vi "DAQ_E_mIO_DIO.get bit.vi"(0 "i ref in":refnum<vi>, 2 "bitIndex":u32, 3 "ms timeout (10000)":i32=10000, 5 "error in (no error)":errorcluster) -> (14 "i ref out":refnum<vi>, 16 "bit":bool, 17 "timed out":bool, 19 "error out":errorcluster)   [LabVIEW 2014, in "DAQ_E_mIO_DIO.lvlib"]
doc: "Gets a bit from a digital input port\n\nLicense Agreement for this software:\n\nCopyright (C)\nGesellschaft für Schwerionenforschung, GSI\nPlanckstr. 1\n64291 Darmstadt\nGermany\n\nContact: D.Beck@gsi.de \n\nThis program is free software; you can redistribute it and/or modify it under the terms of the GNU General Public License as published by the Free Software Foundation; either version 2 of the license, or (at your option) any later version.\n\nThis program is distributed in the hope that it will be useful, but WITHOUT ANY WARRANTY; without even the implied warranty of MERCHANTABILITY or FITNESS FOR A PARTICULAR PURPOSE. See the GNU General License for more details (http://www.gnu.org).\n\nGesellschaft für Schwerionenforschung, GSI\nPlanckstr. 1, 64291 Darmstadt, Germany\nFor all questions and ideas contact: M.Richter@gsi.de, H.Brand@gsi.de or D.Beck@gsi.de.\nLast update: 17-JUN-2004"
uses:
  DAQ_E_mIO_DIO.lvlib
  CSCore/CSSystem/CoreDefs/CoreDefs.error_type.ctl
  CSApplicationBaseClasses/DigiIOBase/DigiIOBase.directionType.ctl
  CSApplicationBaseClasses/DigiIOBase/DigiIOBase.serviceType.ctl
  lib.lib/UtilityLib/UtilityLib.valueStatus.ctl
  <vilib>/DAQmx/read.llb/DAQmx Read (Digital 1D Bool 1Chan 1Samp).vi
  CSCore/CSSystem/CoreLib/CoreLib.lvlib
  CSApplicationBaseClasses/DigiIOBase/DigiIOBase.lvlib
  lib.lib/UtilityLib/UtilityLib.lvlib
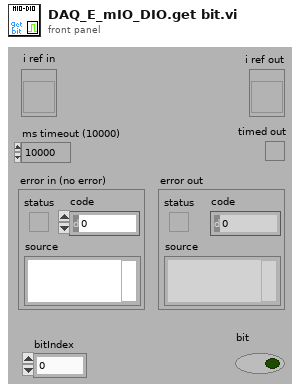
[diagram p1: front panel]
types:
  T1 = typedef "CoreDefs.error_type.ctl" = enum16{"no error", "can't load process", "can't unload process", "process does not exist", "can't install process", "can't remove process", "unknown function", "time out", "can't execute function", "duplicate queue name", "super not found", "caller queue invalid", "can't ping process", "unknown error", "VISA Error", "VISA timeout", "GPIB timeout", "GPIB error", "communication error", "data type mismatch", "can't read data from OPC server", "can't write data to OPC server", "OET error", "function not implemented", "process already exists", "invalid Shared Variable name", "error writing Shared Variable", "error reading Shared Variable", "invalid client name", "corrupt database", "unknown class", "call not authorized", "parameter out of range", "OET timeout: can't get data to modify", "invalid queue name", "requested operation incompatible with current state", "event undefined", "event disabled", "state undefined", "caller is not a friend", "EventBuilder: bad eventID", "EventBuilder: no DAQ devices", "a thread must not stop itself", "UNUSED ELEMENT4", "DiscArchiver: eventData incomplete", "DiscArchiver: eventData does not belong to run", "DiscArchiver: can't open file", "DiscArchiver: can't write to file", "DiscArchiver: available disc space low", "can't acquire semaphore", "error reading data from database", "notifier object is not existing", "can't register process", "can't unregister process", "illegal event type", "object disabled", "object already exists", "can't change state", "Instrument not found", "no connection to remote node", "invalid reference", "N/A", "UNUSED ELEMENT 1", "element not found", "illegal TCP/IP connection detected", "object does not exist", "invalid access ID", "unknown CS system", "invalid privilige", "unsupported data type", "unsupported server type", "IO server already exists", "Shared Variable already exists"}
  T2 = typedef "UtilityLib.lvlib/UtilityLib.valueStatus.ctl" = enum16{"no info available", "stand by/off", "on", "warning", "alarm/malfunction", "not implemented", "user action required", "important information", "system default", "control default", "indicator default", "button default"}
  T3 = typedef "DigiIOBase.lvlib/DigiIOBase.serviceType.ctl" = enum16{"bit", "word"}
  T4 = typedef "DigiIOBase.lvlib/DigiIOBase.directionType.ctl" = enum16{"unknown", "update actual value", "update nominal value", "update both"}
  T5 = typedef "DAQ_E_mIO_DIO.lvlib/DAQ_E_mIO_DIO.i attribute.ctl" = cluster{"DOutChannel":refnum<k21>, "DInChannel":refnum<k21>, "nOfBitsIn":i32, "nOfBitsOut":i32}
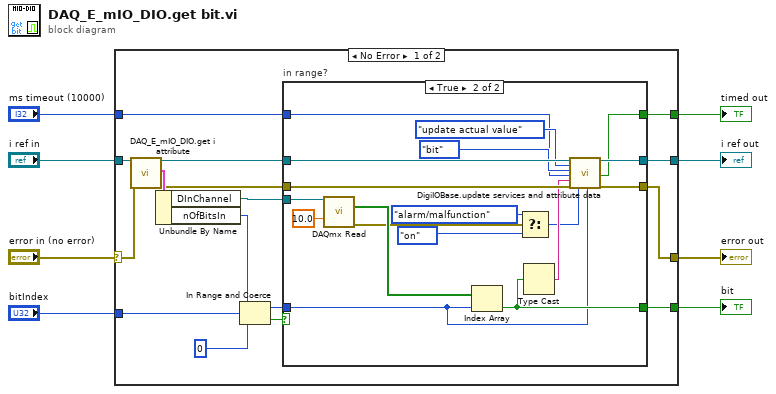
[diagram p0: block diagram]
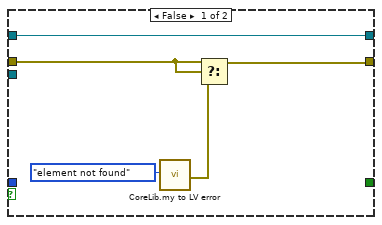
[diagram p2: hidden frame]
diagram:
  n1 = case shown="No Error" "error in (no error)" {
    selector: "error in (no error)" -> [w16 w48]
    tunnel: "i ref in" -> [w17 w49]
    tunnel: [w24 w49] -> w7
    tunnel: [w23 w48] -> w6
    tunnel: "bitIndex" -> [w21 _]
    tunnel: [w18 _] -> w4
    tunnel: "ms timeout (10000)" -> [w10 _]
    tunnel: [w9 _] -> w1
    frame No Error {
      n2 = call "DAQ_E_mIO_DIO.get i attribute.vi"("i ref in"=w17, "error in (no error)"=w16) -> ("i ref out"=w12:refnum<vi>, "i attribute"=w15:T5, "error out"=w13:errorcluster)  [unwired: 15 in]
      n3 = Unbundle By Name(w15) -> ("DInChannel"=w11:refnum<k21>, "nOfBitsIn"=w14:i32)
      n4 = In Range and Coerce(upper limit=w14, x=w21, lower limit=u32 0) -> (coerced(x)=w20:u32, In Range?=w19:bool)
      n5 = case "in range?" shown="True" w19 {
        tunnel: w12 -> [w29 w44]
        tunnel: w13 -> [w28 w42]
        tunnel: [w29 w43] -> w24
        tunnel: [w27 w41] -> w23
        tunnel: w20 -> [_ w30]
        tunnel: [_ w37] -> w18
        tunnel: w11 -> [_ w46]
        tunnel: w10 -> [_ w38]
        tunnel: [_ w35] -> w9
        frame False {
          n6 = call "CoreLib.my to LV error.vi"("ErrorTypes"=CoreDefs.error_type."element not found") -> ("myErrorCluster"=w26:errorcluster)  [unwired: 17 in, 1 out]
          n7 = Select(t=w28, s=w28, f=w26) -> (s? t:f=w27:errorcluster)
        }
        frame True {
          n8 = call-poly <vilib>:"DAQmx Read.vi"("task/channels in"=w46, "timeout"=10.0) -> ("data"=w45:bool[], "error out"=w34:errorcluster)  [unwired: 11 in, 1 out]
          n9 = Index Array(array=w45, index=w30) -> (element=w37:bool)
          n10 = Select(t=UtilityLib.valueStatus."alarm/malfunction", s=w34, f=UtilityLib.valueStatus."on" ("quality")) -> (s? t:f=w31:T2)
          n11 = Type Cast(x=w37) -> (*(type *) &x=w36:string)  [unwired: 1 in]
          n12 = call "DigiIOBase.update services and attribute data.vi"("i ref in"=w44, "direction"=DigiIOBase.directionType."update actual value", "service"=DigiIOBase.serviceType."bit", "ms timeout (10000)"=w38, "value"=w36, "error in (no error)"=w42, "quality"=w31, "index"=w30) -> ("i ref out"=w43:refnum<vi>, "timed out"=w35:bool, "error out"=w41:errorcluster)  [unwired: 9 in]
        }
      }
    }
    frame Error {
    }
  }
  "error out" <- w6
  "i ref out" <- w7
  "bit" <- w4
  "timed out" <- w1
